vi "Error - Fire.vi"(8 "error in (no error)":errorcluster, 11 "UE Data Container":T2) -> (0 "error out":errorcluster)   [LabVIEW 2017]
doc: "Generates Error user event with required parameters"
uses:
  Shared Data/User Events/UE Data Container.ctl
  Controls/Error Data.ctl
panel:
  in  "Data":variant
  in  "Type":T1(ring)
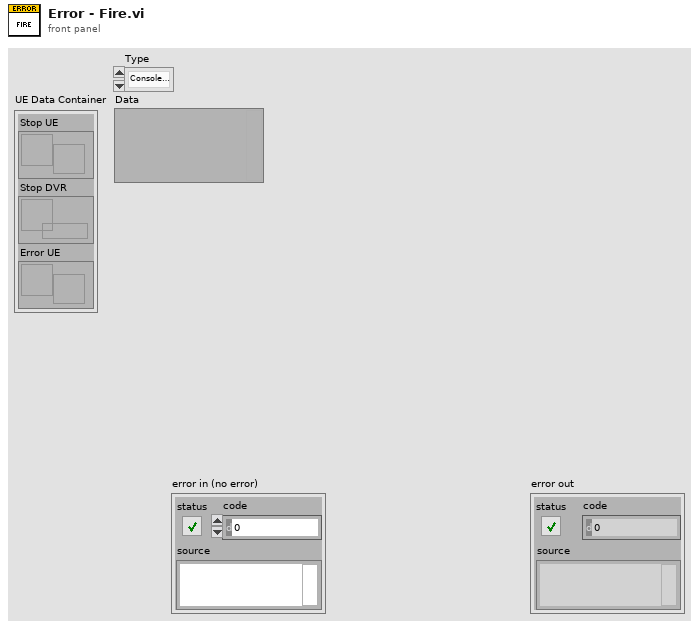
[diagram p1: front panel]
types:
  T1 = enum16{"Console Error", "Sensor Interface IO Error", "Process Step Error"}
  T2 = typedef "UE Data Container.ctl" = cluster{"Stop UE":refnum<user-event>, "Stop DVR":refnum<data-value>, "Error UE":refnum<user-event>}
  T3 = typedef "Error Data.ctl" = cluster{"Type":enum16{"Console Error", "Sensor Interface IO Error", "Process Step Error"}, "Data":variant}
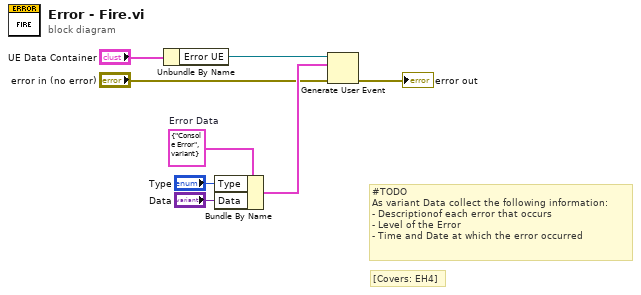
[diagram p0: block diagram]
diagram:
  w6 = T3 {"Type"=enum."Console Error", "Data"=variant}  # Error Data
  # "[Covers: EH4]"
  # "#TODO\nAs variant Data collect the following information:\n- Descriptionof each error that occurs\n- Level of the Error\n- Time and Date at which the error occurred"
  n1 = Unbundle By Name("UE Data Container") -> ("Error UE"=w7:refnum<user-event>)
  n2 = Bundle By Name(cluster=w6, "Type"="Type", "Data"="Data") -> (w3:T3)
  n3 = Generate User Event(user event=w7, event data cluster=w3, error in="error in (no error)") -> (error out=→"error out":errorcluster)  [unwired: 1 in, 1 out]
